vi "New Case tester.vi"() -> ()   [LabVIEW 2020, in "Method Generation.lvlib" / "Setter Generator.lvclass"]
uses:
  Setter Generator.lvclass
  Setter Generator.lvclass/Setter Generator.ctl
panel:
  in  "error in (no error)":errorcluster
  out "error out":errorcluster
  out "output cluster":refnum<class "Setter Generator.lvclass">
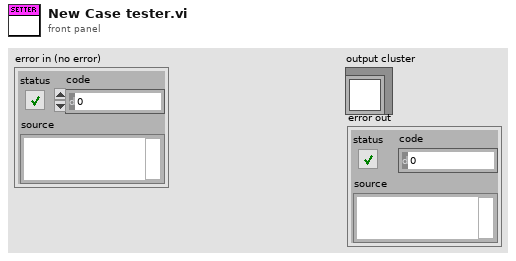
[diagram p1: front panel]
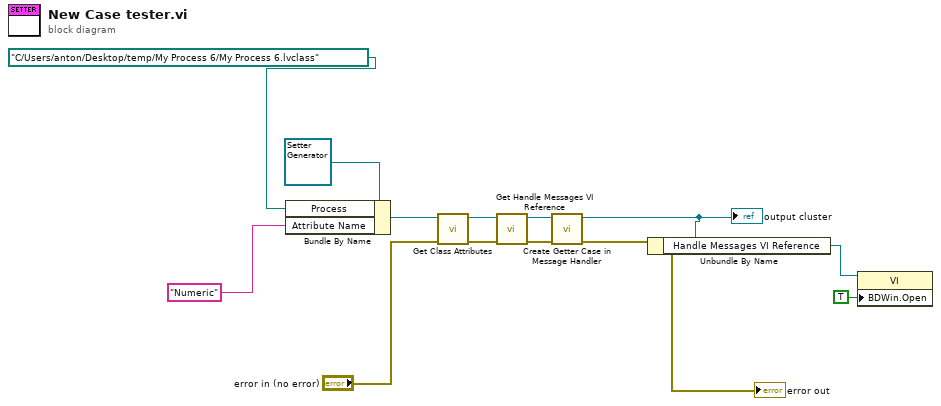
[diagram p0: block diagram]
diagram:
  n1 = Bundle By Name(cluster=refnum<class "Setter Generator.lvclass"> refnum ("New Getter Dialog In"), "Process"=path "C:/Users/anton/Desktop/temp/My Process 6/My Process 6.lvclass" ("class path"), "Attribute Name"="Numeric") -> (w4:refnum<class "Setter Generator.lvclass">)
  n2 = call "Get Class Attributes.vi"("error in (no error)"="error in (no error)", "Setter Generator In"=w4) -> ("error out"=w1:errorcluster, "Setter Generator Out"=w3:refnum<class "Setter Generator.lvclass">)  [unwired: 8 in]
  n3 = call "Get Handle Messages VI Reference.vi"("error in (no error)"=w1, "Setter Generator In"=w3) -> ("error out"=w8:errorcluster, "Setter Generator Out"=w10:refnum<class "Setter Generator.lvclass">)  [unwired: 8 in]
  n4 = call "Create Getter Case in Message Handler.vi"("error in (no error)"=w8, "Setter Generator In"=w10) -> ("error out"=→"error out":errorcluster, "Setter Generator Out"=w7:refnum<class "Setter Generator.lvclass">)  [unwired: 8 in]
  "output cluster" <- w7
  n5 = Unbundle By Name(w7) -> ("Handle Messages VI Reference"=w6:refnum<vi>)
  n6 = property class="VI"(reference=w6, "BDWin.Open"=TRUE ("Block Diagram Window:Open")) -> ()  [unwired: 1 in, 2 out]
